vi "Set Scaling Equation.vi"(0 "session in":refnum<k21>, 1 "serial number":string, 2 "password":string, 5 "physical channel":refnum<k21>="$DefaultPhysChans", 7 "equation":string, 11 "error in (no error)":errorcluster) -> (4 "session out":refnum<k21>, 6 "physical channel out":refnum<k21>, 15 "error out":errorcluster)   [LabVIEW 2020, in "SLSC.lvlib"]
doc: "Sets the scaling equation for a user-defined scale."
uses:
  <vilib>/SLSC/SLSC.lvlib
  nislsclvapi.dll
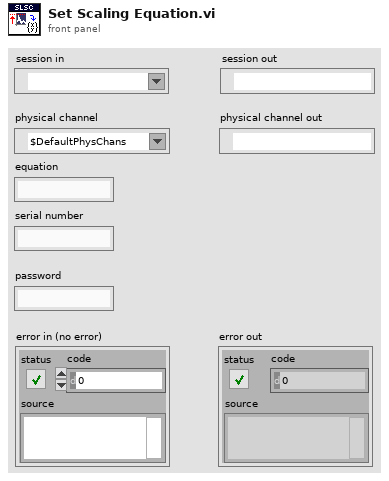
[diagram p1: front panel]
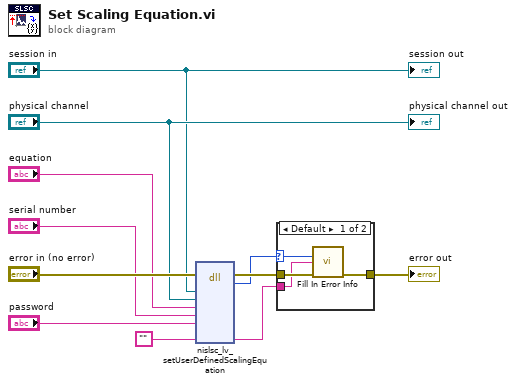
[diagram p0: block diagram]
diagram:
  n1 = dll-call lib="nislsclvapi.*" fn="nislsc_lv_setUserDefinedScalingEquation"(error in="error in (no error)", "session"="session in", "physical channel"="physical channel", "equation"="equation", "serialNum"="serial number", "password"="password", "extendedErrorInfo"="") -> (error out=w4:errorcluster, "return type"=w1:i32, "extendedErrorInfo"=w3:string)  [unwired: 9 in, 1 out]
  n2 = case shown="Default" w1 {
    selector: w1 -> [w12 _]
    tunnel: w3 -> [w13 _]
    tunnel: w4 -> [w15 w16]
    tunnel: [w14 w16] -> w2
    frame Default {
      n3 = call <vilib>:"Fill In Error Info.vi"("status code"=w12, "extended error info"=w13, "error in"=w15) -> ("error out"=w14:errorcluster)  [unwired: 12 in]
    }
    frame 0 {
    }
  }
  "error out" <- w2
  "session out" <- "session in"
  "physical channel out" <- "physical channel"
